vi "TestWriteFromMote.vi"() -> ()   [LabVIEW 2010]
uses:
  <vilib>/picture/picture.llb/Draw True-Color Pixmap.vi
panel:
  out "Waveform Chart":i32(graph)
  in  "Dummy":i16
  out "Bytes written":i32
  out "Packet Payload":string
  in  "Enable Write":bool=TRUE
  in  "Port Number":i32=9002
  out "KTH  Automatic Control \nTemplates. Write to the SerialForwarder":picture
  # "Communication control"
  # "Communication results"
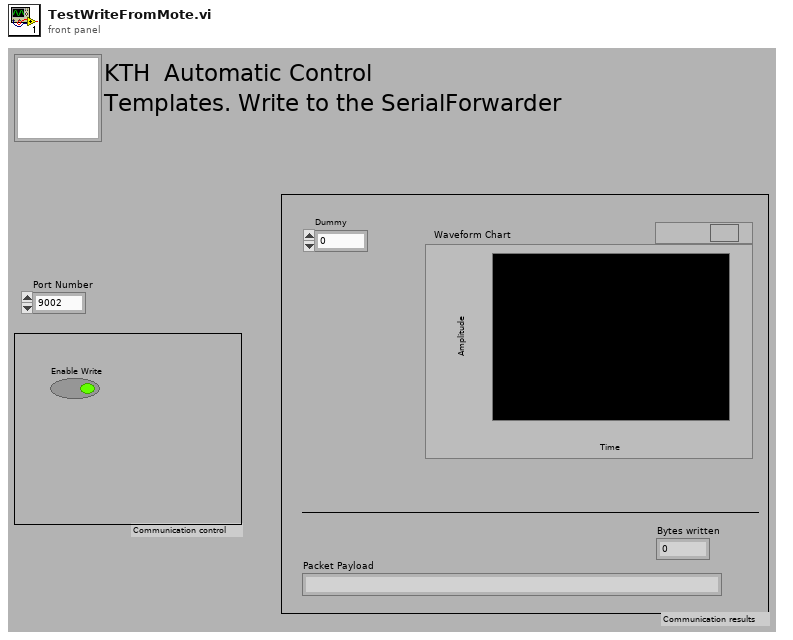
[diagram p1: front panel]
types:
  T1 = typedef "imagedata.ctl" = cluster{"image type":i32, "image depth":i32, "image":u8[], "mask":u8[], "colors":u32[], "Rectangle":cluster{"left":i16, "top":i16, "right":i16, "bottom":i16}}
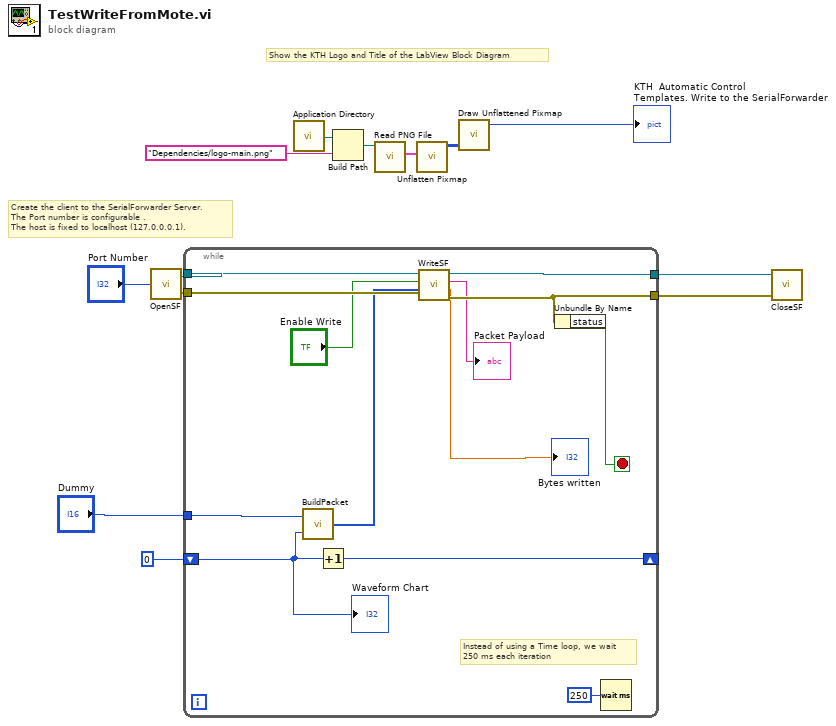
[diagram p0: block diagram]
diagram:
  # "Create the client to the SerialForwarder Server.\nThe Port number is configurable . \nThe host is fixed to localhost (127.0.0.0.1)."
  # "Show the KTH Logo and Title of the LabView Block Diagram"
  n1 = call "OpenSF.vi"("Port Number"="Port Number") -> ("error out"=w12:errorcluster, "connection ID"=w13:refnum<k5>)
  n2 = while {
    tunnel: w13 -> [w25]
    tunnel: w12 -> [w26]
    tunnel: [w24] -> w11
    tunnel: [w22] -> w10
    tunnel: "Dummy" -> [w16]
    shift-right: [w15] -> _
    shift-left: 0 -> [w14]
    stop <- w23 stop-if-true
    # "Instead of using a Time loop, we wait \n250 ms each iteration"
    n3 = call "BuildPacket.vi"("Counter"=w14, "Dummy"=w16) -> ("PacketArray"=w17:i32[])
    n4 = Increment(x=w14) -> (x+1=w15:i32)
    n5 = call "WriteSF.vi"("error in"=w26, "packet"=w17, "Enablle write"="Enable Write", "connection ID"=w25) -> ("error out"=w22:errorcluster, "Bytes written to SF"=→"Bytes written":dbl, "Packet String"=→"Packet Payload":string, "connection ID out"=w24:refnum<k5>)
    n6 = Unbundle By Name(w22) -> ("status"=w23:bool)
    n7 = Wait (ms)(milliseconds to wait=u32 250) -> ()  [unwired: 1 out]
    "Waveform Chart" <- w14
  }
  n8 = call <vilib>:"Application Directory.vi"() -> ("Application Directory"=w5:path)
  n9 = Build Path(base path=w5, name or relative path="Dependencies/logo-main.png") -> (appended path=w6:path)
  n10 = call <vilib>:"Read PNG File.vi"("path to PNG file"=w6) -> ("image data"=w9:T1)  [unwired: 8 in, 2 out]
  n11 = call <vilib>:"Unflatten Pixmap.vi"("image data"=w9) -> ("24-bit pixmap"=w8:u32[][])  [unwired: 4 in, 6 out]
  n12 = call-poly <vilib>:"Draw Unflattened Pixmap.vi"("data (RGB format)"=w8) -> ("new picture"=→"KTH  Automatic Control \nTemplates. Write to the SerialForwarder":picture)  [unwired: 8 in]
  n13 = call "CloseSF.vi"("error out"=w10, "connection ID"=w11) -> ()  [unwired: 1 in]
